vi "Double move fwd PID.vi"(0 "Distance":dbl, 1 "Gains":T1={"proportional gain (Kc)"=1.0, "integral time (Ti, min)"=0.01, "derivative time (Td, min)"=0.0} {"derivative time (Td, min)" format="%.3f"; "integral time (Ti, min)" format="%.3f"; "proportional gain (Kc)" format="%.3f"}, 3 "Range":cluster{"output high":dbl, "output low":dbl}={"output high"=1.0, "output low"=0.0} {"output low" format="%.2f"; "output high" format="%.2f"}, 5 "Encoder Left":dbl, 7 "Reset Rate":bool, 9 "Encoder Right":dbl, 11 "Precision":dbl=0.5 format="%#_13g", 12 "Loop Timer":i32=20, 14 "Time to stop":i32=300) -> (4 "PWM Left":dbl=0.5 format="%#_13g", 6 "PWM Right":dbl=0.5 format="%#_13g", 15 "Both finished?":bool)   [LabVIEW 2017]
panel:
  # "Time to stop - Tempo que o encoder deve retornar um valor dentro do range da precision para a função considerar que o sistema está parado.\n\nDistance - Setpoint em unidades do encoder.\n\nLoop Timer - Tempo de iteração do loop em que a função está.\n\nPrecision - Range que a função considera \"close enough\" ao setpoint.\n\nEncoder Right - Valor atual do encoder da direita.\n\nEncoder Left - Valor atual do encoder da esquerda\n\nRate limit - Limite de aceleração/desaceleração do sistema.\n\nGains - Ganhos do PID.\n\nRange - limite superior e inferior do PID.\n\nSoft Start - constante que aumenta ou diminui o tempo de aceleração no início do movimento"
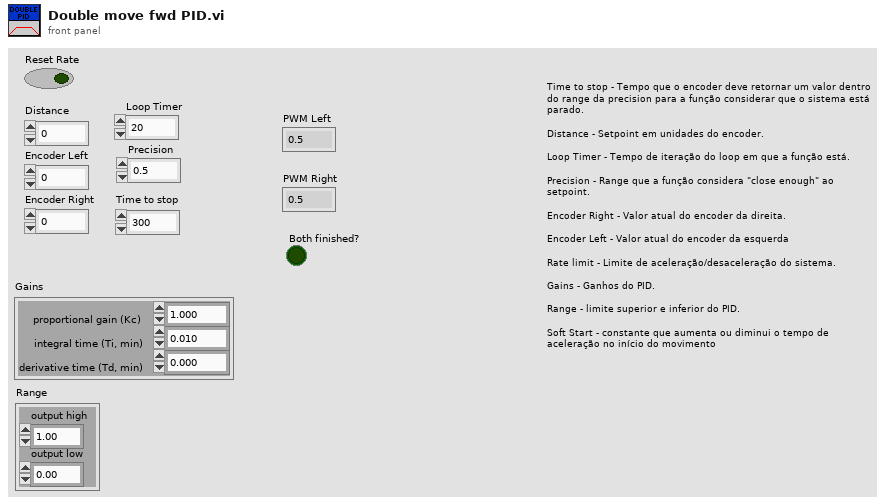
[diagram p1: front panel]
types:
  T1 = cluster{"proportional gain (Kc)":dbl, "integral time (Ti, min)":dbl, "derivative time (Td, min)":dbl}
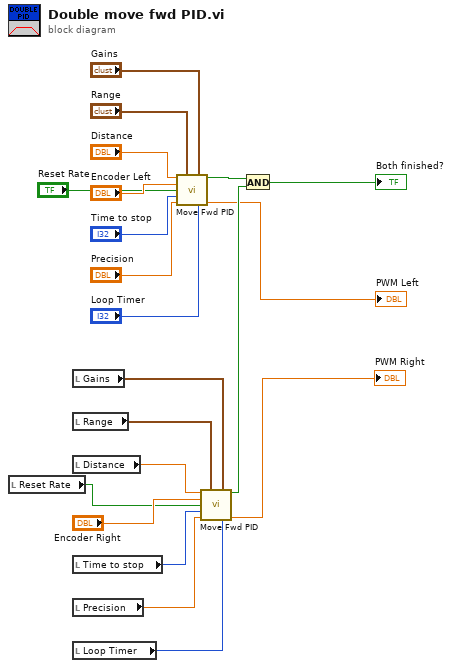
[diagram p0: block diagram]
diagram:
  n1 = local read "Reset Rate"() -> (w1:bool)
  n2 = local read "Gains"() -> (w13:T1)
  n3 = local read "Range"() -> (w12:cluster{"output high":dbl, "output low":dbl})
  n4 = local read "Distance"() -> (w11:dbl)
  n5 = local read "Time to stop"() -> (w10:i32)
  n6 = local read "Precision"() -> (w9:dbl)
  n7 = local read "Loop Timer"() -> (w8:i32)
  n8 = call "Move Fwd PID.vi"("Distance"="Distance", "Range"="Range", "Gains"="Gains", "Encoder Count"="Encoder Left", "Reset Rate"="Reset Rate", "Time to stop"="Time to stop", "Precision"="Precision", "Loop Timer"="Loop Timer") -> ("Finished?"=w7:bool, "Output"=→"PWM Left":dbl)  [unwired: 6 in]
  n9 = call "Move Fwd PID.vi"("Distance"=w11, "Range"=w12, "Gains"=w13, "Encoder Count"="Encoder Right", "Reset Rate"=w1, "Time to stop"=w10, "Precision"=w9, "Loop Timer"=w8) -> ("Finished?"=w6:bool, "Output"=→"PWM Right":dbl)  [unwired: 6 in]
  n10 = And(x=w7, y=w6) -> (x .and. y?=→"Both finished?":bool)
